vi "Handle HTTP Response.vi"(5 "Headers":string, 7 "Body":string, 11 "error in (no error)":errorcluster) -> (15 "error out":errorcluster)   [LabVIEW 2023, in "VolatusSeq.lvlib" / "State.lvclass"]
uses:
  State.lvclass
  State.lvclass/State.ctl
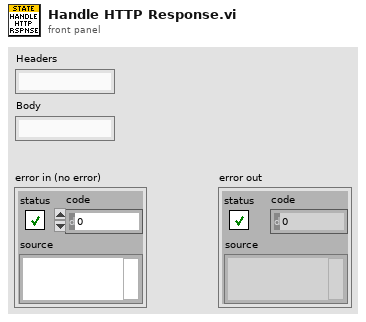
[diagram p1: front panel]
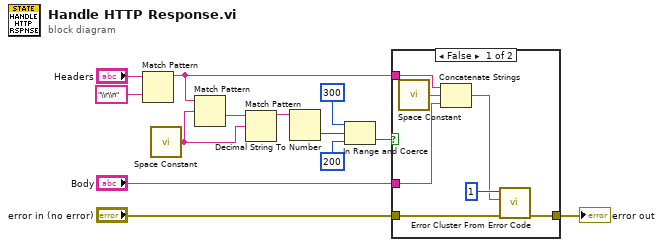
[diagram p0: block diagram]
diagram:
  n1 = Match Pattern(string="Headers", regular expression="\\r\\n") -> (before substring=w2:string)  [unwired: 1 in, 3 out]
  n2 = call <vilib>:"Space Constant.vi"() -> ("String"=w10:string)
  n3 = Match Pattern(string=w2, regular expression=w10) -> (after substring=w11:string)  [unwired: 1 in, 3 out]
  n4 = Match Pattern(string=w11, regular expression=w10) -> (before substring=w9:string)  [unwired: 1 in, 3 out]
  n5 = Decimal String To Number(string=w9) -> (number=w8:i32)  [unwired: 2 in, 1 out]
  n6 = In Range and Coerce(upper limit=300, x=w8, lower limit=200 ("upper limit")) -> (In Range?=w5:bool)  [unwired: 1 out]
  n7 = case shown="False" w5 {
    tunnel: "error in (no error)" -> [w20 w21]
    tunnel: "Body" -> [w15 _]
    tunnel: w2 -> [w17 _]
    tunnel: [w19 w21] -> w1
    frame False {
      n8 = call <vilib>:"Space Constant.vi"() -> ("String"=w16:string)
      n9 = Concatenate Strings(w17, w16, w15) -> (w14:string)
      n10 = call <vilib>:"Error Cluster From Error Code.vi"("error in (no error)"=w20, "error message (\"\")"=w14, "error code (0)"=1) -> ("error out"=w19:errorcluster)  [unwired: 6 in]
    }
    frame True {
    }
  }
  "error out" <- w1
